vi "GV_Undo_add.vi"(8 "error in (no error)":errorcluster, 9 "ZoomEvent":T1, 11 "Gviewer in":refnum<class "Gviewer.lvclass">) -> (0 "error out":errorcluster, 3 "Gviewer out":refnum<class "Gviewer.lvclass">)   [LabVIEW 2020, in "Sgraph_lib_V1.lvlib" / "Gviewer.lvclass"]
doc: "Add one undo event to the undo memory"
uses:
  Gviewer.lvclass
  controls/Typedef_ZoomEvent.ctl
  controls/Typedef_Live.ctl
  controls/Typedef_SelProperties.ctl
  controls/Typedef_LineType.ctl
  Gviewer.lvclass/Gviewer.ctl
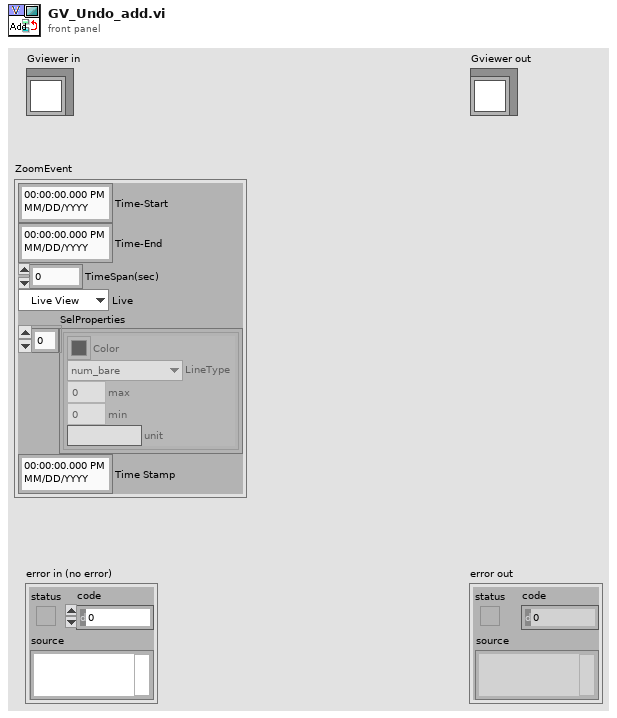
[diagram p1: front panel]
types:
  T1 = typedef "Sgraph_lib_V1.lvlib/Gviewer.lvclass/Typedef_ZoomEvent.ctl" = cluster{"Time-Start":timestamp, "Time-End":timestamp, "TimeSpan(sec)":dbl, "Live":T2, "SelProperties":T3[], "Time Stamp":timestamp}
  T2 = typedef "Sgraph_lib_V1.lvlib/Gviewer.lvclass/Typedef_Live.ctl" = enum16{"Live View", "Freeze"}
  T3 = typedef "Sgraph_lib_V1.lvlib/Gviewer.lvclass/Typedef_SelProperties.ctl" = cluster{"Color":u32, "LineType":T4, "max":dbl, "min":dbl, "unit":string}
  T4 = typedef "Sgraph_lib_V1.lvlib/Gviewer.lvclass/Typedef_LineType.ctl" = enum16{"num_bare", "num_MinMax_Area", "num_MinMax_Lines", "num_MinMax_Forfor", "num_Max_Area", "num_Max_Line", "num_Max_Forfor", "num_Min_Area", "num_Min_Line", "num_Min_Fosfor", "Boolean_Line_01", "Boolean_Area_01", "Boolean_Fosfor_01", "Boolean_Line_TF", "Boolean_Area_TF", "Boolean_Fosfor_TF", "Boolean_OnOff_Line", "Boolean_OnOff_Area", "Boolean_OnOff_Fosfor", "Boolean_spare", "StringEvent_Line", "StringEvent_TimeLine"}
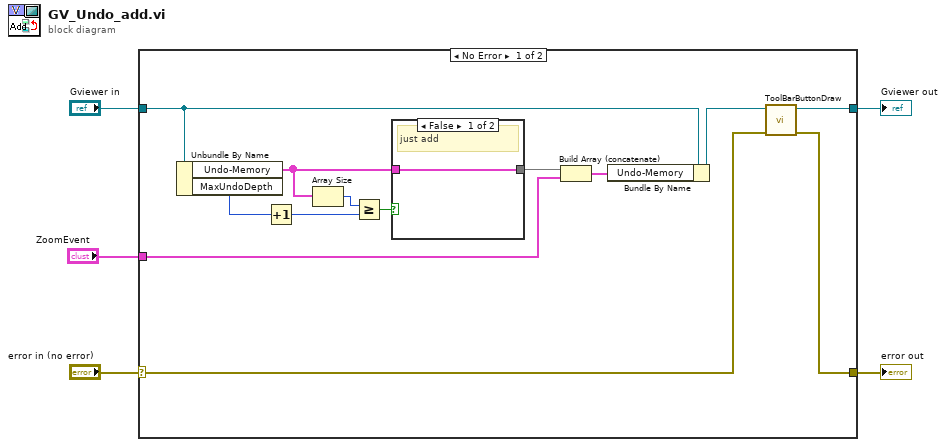
[diagram p0: block diagram]
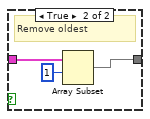
[diagram p2: hidden frame]
diagram:
  n1 = case shown="No Error" "error in (no error)" {
    selector: "error in (no error)" -> [w7 w24]
    tunnel: [w6 w24] -> w4
    tunnel: [w8 w23] -> w2
    tunnel: "Gviewer in" -> [w11 w23]
    tunnel: "ZoomEvent" -> [w13 _]
    frame No Error {
      n2 = Unbundle By Name(w11) -> ("Undo-Memory"=w15:T1[], "MaxUndoDepth"=w17:i32)
      n3 = Increment(x=w17) -> (x+1=w10:i32)
      n4 = Array Size(array=w15) -> (size(s)=w18:i32)
      n5 = Greater Or Equal?(x=w18, y=w10) -> (x >= y?=w16:bool)
      n6 = case shown="False" w16 {
        tunnel: w15 -> [w19 w22]
        tunnel: [w19 w20] -> w14
        frame False {
          # "just add"
        }
        frame True {
          # "Remove oldest"
          n7 = Array Subset(array=w22, index=1) -> (w20:T1[])  [unwired: 1 in]
        }
      }
      n8 = Build Array (concatenate)(w14, w13) -> (w12:T1[])
      n9 = Bundle By Name(cluster=w11, "Undo-Memory"=w12) -> (w9:refnum<class "Gviewer.lvclass">)
      n10 = call "ToolBarButtonDraw.vi"("error in (no error)"=w7, "Gviewer in"=w9) -> ("error out"=w6:errorcluster, "Gviewer out"=w8:refnum<class "Gviewer.lvclass">)  [unwired: 8 in]
    }
    frame Error {
    }
  }
  "error out" <- w4
  "Gviewer out" <- w2
